vi "MerweScSigPts_GetWm_Single.vi"(9 "Element":i32, 11 "MerweScaledSigmaPts":T1) -> (3 "Mw_Value":dbl)   [LabVIEW 2019, in "Trajectory_Library.lvlib"]
doc: "Returns an element of the weight for each sigma point for the mean.\n \nInputs:\n - MerweScaledSigmaPts -- data cluster\n - element -- Element of vector to return.\n\nOutputs:\n - Wm_Value -- the element i's weight for the mean."
uses:
  Trajectory_Library.lvlib
  TypeDef/MERWE_SCALED_SIGMA_PTS.ctl
  <vilib>/Analysis/Matrix/Datatypes/RealMatrix.ctl
  <vilib>/Analysis/Matrix/NI_Matrix.lvlib
panel:
  # "<?, 1>"
  # "<?, 1>"
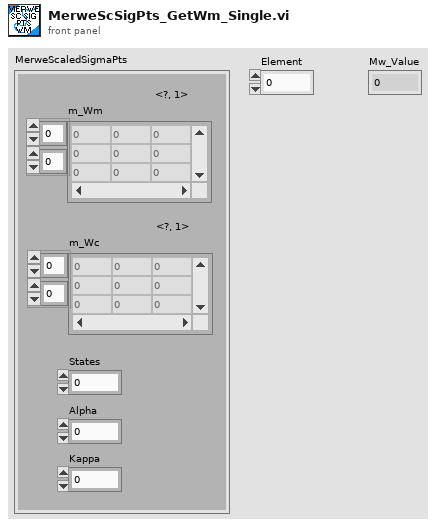
[diagram p1: front panel]
types:
  T1 = typedef "Trajectory_Library.lvlib/MERWE_SCALED_SIGMA_PTS.ctl" = cluster{"m_Wm":T2, "States":i32, "Alpha":dbl, "m_Wc":T2, "Kappa":i32}
  T2 = typedef "NI_Matrix.lvlib/RealMatrix.ctl" = dbl[][]
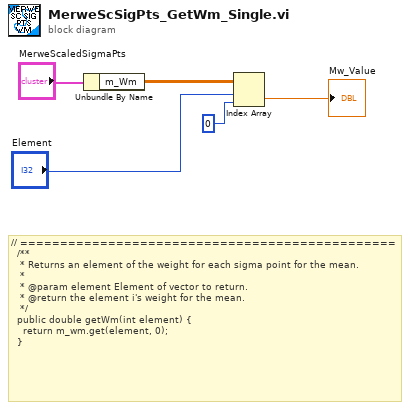
[diagram p0: block diagram]
diagram:
  # "// ===============================================\n  /**\n   * Returns an element of the weight for each sigma point for the mean.\n   *\n   * @param element Element of vector to return.\n   * @return the element i's weight for the mean.\n   */\n  public double getWm(int element) {\n    return m_wm.get(element, 0);\n  }"
  n1 = Unbundle By Name("MerweScaledSigmaPts") -> ("m_Wm"=w1:T2)
  n2 = Index Array(array=w1, index (row)="Element", index (col)=0) -> (element=→"Mw_Value":dbl)
